vi "Set Rep Rounds.vi"(8 "error in (no error)":errorcluster, 10 "Rep Rounds":u32, 11 "Map in":refnum<class "Map.lvclass">) -> (0 "error out":errorcluster, 3 "Map out":refnum<class "Map.lvclass">)   [LabVIEW 2020, in "SquareBattle.lvlib" / "Map.lvclass"]
uses:
  Map.lvclass
  Map.lvclass/Map.ctl
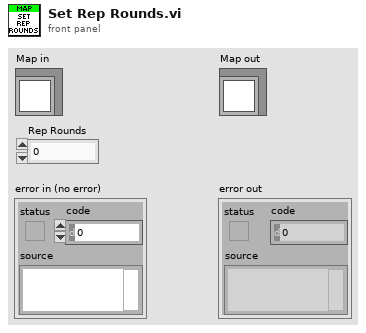
[diagram p1: front panel]
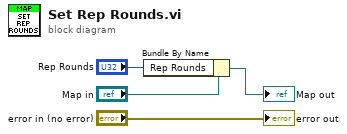
[diagram p0: block diagram]
diagram:
  n1 = Bundle By Name(cluster="Map in", "Rep Rounds"="Rep Rounds") -> (→"Map out":refnum<class "Map.lvclass">)
  "error out" <- "error in (no error)"
